vi "ZeroGyro.vi"(8 "error in":errorcluster) -> (0 "error out":errorcluster)   [LabVIEW 2016]
uses:
  NavX Library/NavX/NavX Library.lvlib
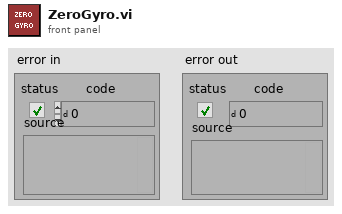
[diagram p1: front panel]
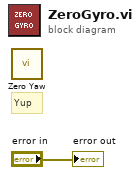
[diagram p0: block diagram]
diagram:
  # "Yup"
  n1 = call "Zero Yaw.vi"() -> ()  [unwired: 12 in]
  "error out" <- "error in"
